vi "Main_FPGA.vi"() -> ()   [LabVIEW 2015]
uses:
  <vilib>/LabVIEW Targets/FPGA/cRIO/shared/nicrio_ModuleControls/nicrio_cRIO-9232_ConfigModeRing.ctl
  <vilib>/rvi/Emulation/niFpgaGetClockAttributes.vi
  <vilib>/rvi/Emulation/niFpgaSctlEmulationGetInTimedLoop.vi
  <vilib>/rvi/Emulation/niFpgaEmulationReportErrorSimple.vi
  <vilib>/rvi/Emulation/niFpgaProcessEmulError.vi
  <vilib>/rvi/eio/common/nirviEmuTemplateMethod_errors.vi
  <vilib>/rvi/interface/RandomDataEmulation/niFpgaRandomDataHandleErrors.vi
  <vilib>/rvi/Emulation/niFpgaCriticalErrorInLSC.vi
  <vilib>/eio/EIONode/EIONode.xnode
  <vilib>/rvi/DataTransferAndStorage/Container/XNode/niFpgaContainer.xnode
  <vilib>/rvi/interface/RandomDataEmulation/nirviRandomDataFpgaReadWriteTemplate.vi
  <vilib>/addons/InsightCM/Devices/Shared/AcquireBOP/FPGA/subVIs/VibAPI/BOP_VibAPI_6.lvlib
panel:
  out "Loop delay (us)":u32
  out "Chassis Temperature":sgl
  in  "Custom Scale Intercept":sgl[](array[numeric])=[0.0, 0.0, 0.0, 0.0, 0.0, 0.0, 0.0, 0.0, 0.0, 0.0, 0.0, 0.0, 0.0, 0.0, 0.0, 0.0, 0.0, 0.0, 0.0, 0.0, 0.0, 0.0, 0.0, 0.0]
  out "FPGA Error":errorcluster
  out "Finished":bool
  in  "Stop":bool
  out "Module Underflow":bool
  out "DMA FIFO Full":bool
  out "Chan Count":bool
  out "Acq Loop Ticks":u32
  out "Short Circuit Chan Array":bool[](array[boolean])
  out "Open Loop Chan Array":bool[](array[boolean])
  out "First Read":bool
  in  "Total Avail Channels":i32=4
  in  "Data Rate [S/s]":u32=1280
  in  "Custom Scale Slope":sgl[](array[numeric])=[0.0, 0.0, 0.0, 0.0, 0.0, 0.0, 0.0, 0.0, 0.0, 0.0, 0.0, 0.0, 0.0, 0.0, 0.0, 0.0, 0.0, 0.0, 0.0, 0.0, 0.0, 0.0, 0.0, 0.0]
  in  "Acquisition Type":enum16{"Finite Samples", "Continuous Samples"}(ring)
  in  "Samps per Chan [Finite]":i32=5120
  in  "Input Config Array":T1[](array[typedef])=[0, 0, 0, 0, 0, 0, 0, 0, 0, 0, 0, 0, 0, 0, 0, 0, 0, 0, 0, 0, 0, 1, 1, 1] items=["AC Coupled", "DC Coupled", "IEPE AC Coupled"]
  in  "Number of Modules":i16=1
  in  "Enable Chan Array":bool[](array[boolean])=[FALSE, FALSE, FALSE, FALSE, FALSE, FALSE, FALSE, FALSE, FALSE, FALSE, FALSE, FALSE, FALSE, FALSE, FALSE, FALSE, FALSE, FALSE, FALSE, FALSE, FALSE, FALSE, FALSE, FALSE]
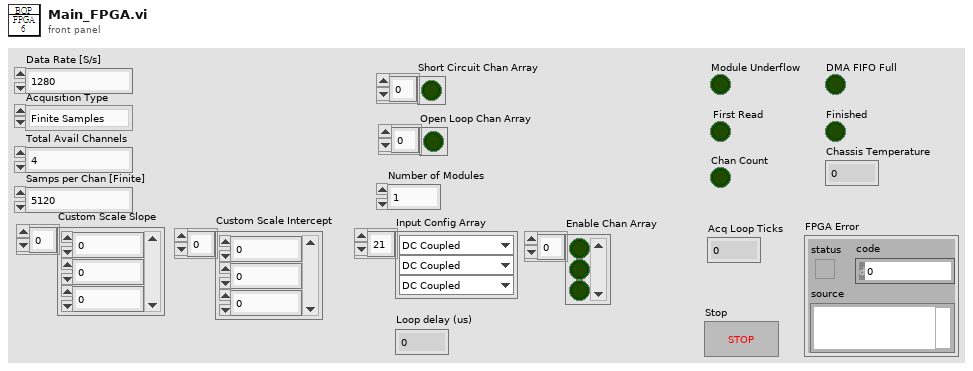
[diagram p1: front panel]
types:
  T1 = typedef "nicrio_cRIO-9232_ConfigModeRing.ctl" = u8
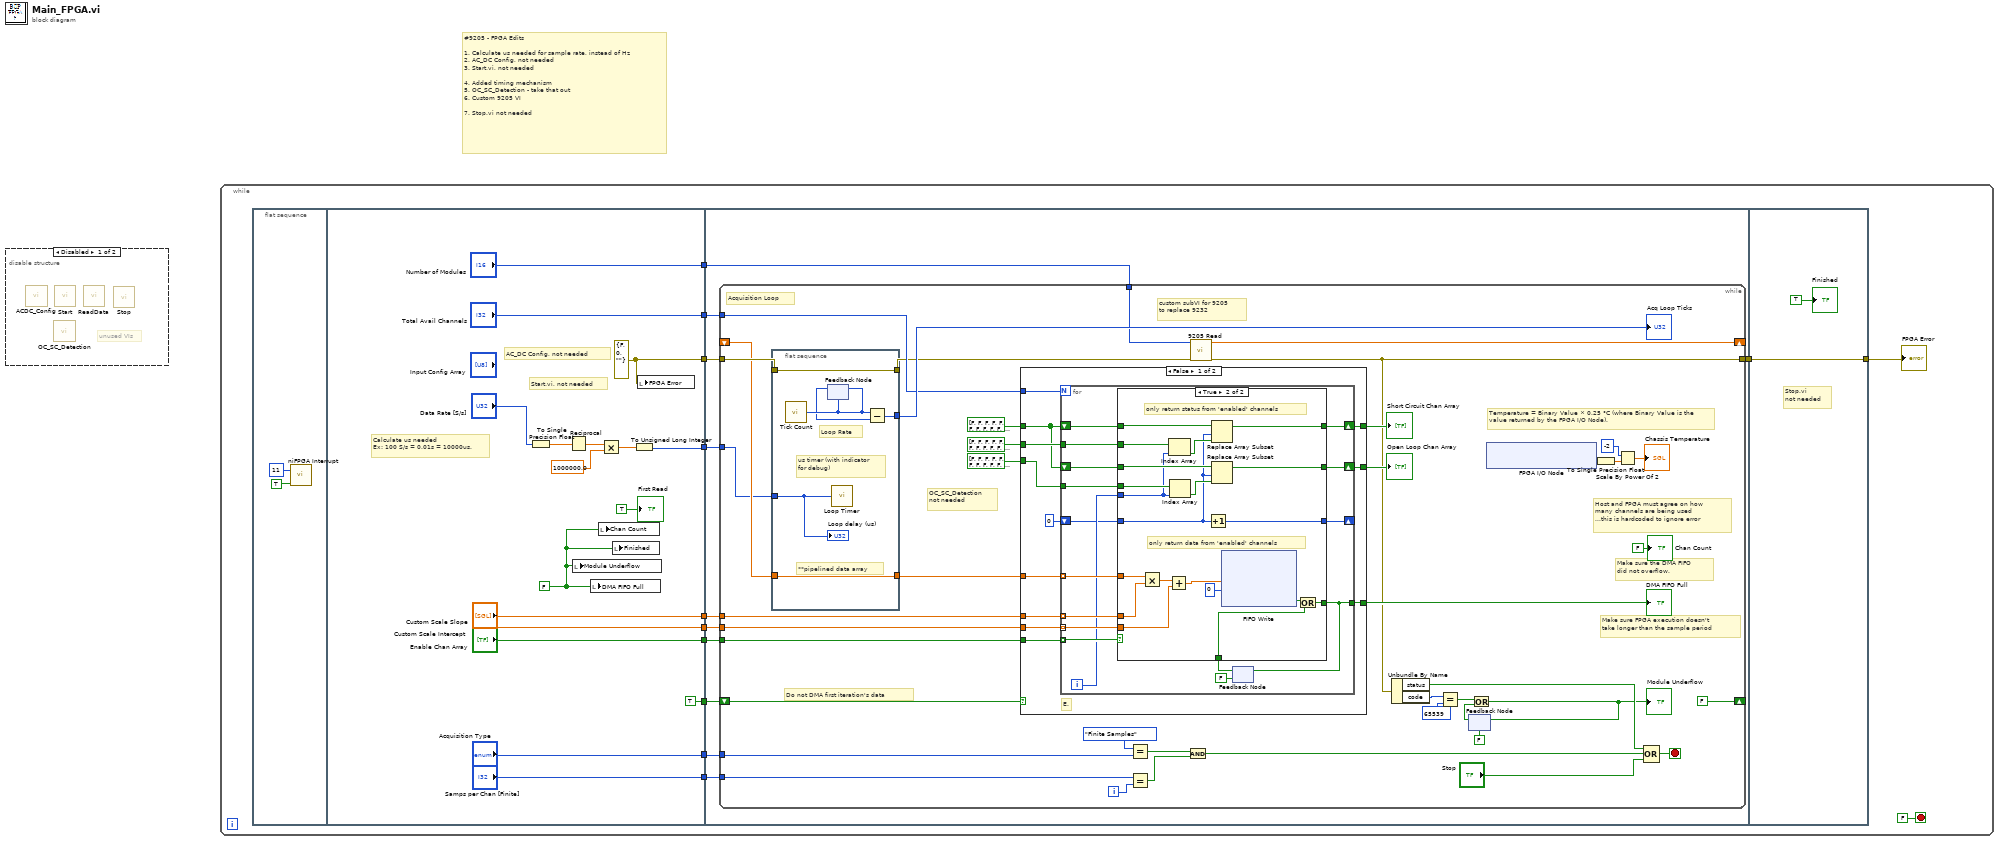
[diagram p0: block diagram]
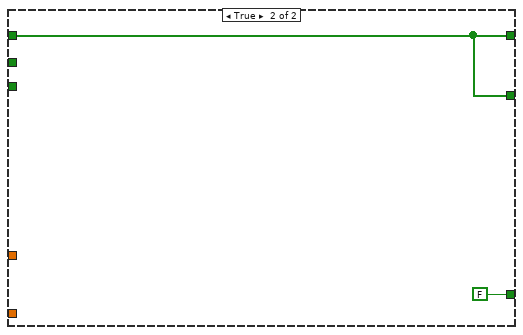
[diagram p4: hidden frame]
diagram:
  # "#9205 - FPGA Edits\n\n1. Calculate us needed for sample rate, instead of Hz\n2. AC_DC Config, not needed\n3. Start.vi, not needed\n\n4. Added timing mechanism\n5. OC_SC_Detection - take that out\n6. Custom 9205 VI\n\n7. Stop.vi not needed"
  n1 = disable-structure shown="Disabled" {
    frame Disabled {
      # "unused VIs"
      n2 = call <vilib>:"ACDC_Config.vi"() -> ()  [unwired: 11 in, 1 out]
      n3 = call <vilib>:"OC_SC_Detection.vi"() -> ()  [unwired: 10 in, 2 out]
      n4 = call <vilib>:"Start.vi"() -> ()  [unwired: 11 in, 1 out]
      n5 = call <vilib>:"ReadData.vi"() -> ()  [unwired: 10 in, 2 out]
      n6 = call <vilib>:"Stop.vi"() -> ()  [unwired: 11 in, 1 out]
    }
    frame Enabled {
    }
  }
  n7 = while {
    stop <- FALSE stop-if-true
    n8 = flat-sequence {
      tunnel: [w22] -> w12
      tunnel: ["Custom Scale Slope"] -> w11
      tunnel: ["Acquisition Type"] -> w10
      tunnel: ["Samps per Chan [Finite]"] -> w9
      tunnel: ["Total Avail Channels"] -> w8
      tunnel: [TRUE ("t")] -> w7
      tunnel: ["Number of Modules"] -> w5
      tunnel: ["Enable Chan Array"] -> w4
      tunnel: ["Custom Scale Intercept"] -> w2
      tunnel: [w16] -> w1
      tunnel: w12 -> [w42]
      tunnel: w11 -> [w41]
      tunnel: w10 -> [w39]
      tunnel: w9 -> [w38]
      tunnel: w8 -> [w43]
      tunnel: w7 -> [w40]
      tunnel: [w37] -> w6
      tunnel: w5 -> [w36]
      tunnel: w4 -> [w35]
      tunnel: w2 -> [w34]
      tunnel: w1 -> [w33]
      tunnel: w6 -> [w146]
      tunnel: [w146] -> w3
      frame #0 {
        n9 = call <vilib>:"niFPGA Interrupt.vi"("Wait Until Cleared (F)"=TRUE ("Wait Until Cleared"), "IRQ Number (0)"=u8 11 ("IRQ Number")) -> ()  [unwired: 1 in]
      }
      frame #1 {
        w22 = errorcluster {"status"=FALSE, "code"=0, "source"=""} ("FPGA Error")
        w27 = FALSE ("Module Underflow")
        # "Start.vi, not needed"
        # "AC_DC Config, not needed"
        # "Calculate us needed\nEx: 100 S/s = 0.01s = 10000us."
        n10 = To Single Precision Float(number="Data Rate [S/s]") -> (single precision float=w19:sgl)
        n11 = Reciprocal(x=w19) -> (1/x=w21:sgl)
        n12 = local write "Module Underflow"(w27) -> ()
        n13 = local write "DMA FIFO Full"(w27) -> ()
        n14 = local write "Chan Count"(w27) -> ()
        n15 = Multiply(x=w21, y=sgl 1000000.0) -> (x*y=w17:sgl)
        n16 = local write "Finished"(w27) -> ()
        n17 = To Unsigned Long Integer(number=w17) -> (unsigned 32bit integer=w16:u32)
        n18 = local write "FPGA Error"(w22) -> ()
        "First Read" <- TRUE ("First Read")
      }
      frame #2 {
        n19 = while {
          tunnel: w42 -> [w79]
          tunnel: [w46] -> w37
          tunnel: w39 -> [w81]
          tunnel: w38 -> [w80]
          shift-right: [w44] -> _
          shift-left: _ -> [w77]
          tunnel: w43 -> [w61]
          tunnel: w41 -> [w60]
          shift-right: [FALSE ("t")] -> _
          shift-left: w40 -> [w64]
          tunnel: w36 -> [w45]
          tunnel: w35 -> [w59]
          tunnel: w34 -> [w58]
          tunnel: w33 -> [w50]
          i -> [w75]
          stop <- w84 stop-if-true
          # "custom subVI for 9205\nto replace 9232"
          # "OC_SC_Detection\nnot needed"
          # "Temperature = Binary Value × 0.25 °C (where Binary Value is the value returned by the FPGA I/O Node)."
          # "Do not DMA first iteration's data"
          # "Acquisition Loop"
          # "Host and FPGA must agree on how \nmany channels are being used\n...this is hardcoded to ignore error"
          # "Make sure the DMA FIFO\ndid not overflow."
          # "Make sure FPGA execution doesn't\ntake longer than the sample period"
          n20 = flat-sequence {
            tunnel: [w145] -> w47
            tunnel: w79 -> [w145]
            tunnel: [w142] -> w78
            tunnel: w77 -> [w141]
            tunnel: [w141] -> w62
            tunnel: w50 -> [w140]
            frame #0 {
              # "us timer (with indicator\nfor debug)"
              # "**pipelined data array"
              # "Loop Rate"
              n21 = call "Tick Count"() -> ("Tick Count(Ticks)"=w144:u32)
              n22 = feedback-in #1(w144) -> ()
              n23 = feedback #1(w144) -> (w143:u32)
              n24 = call "Loop Timer"("Count(uSec)"=w140) -> ()  [unwired: 1 out]
              n25 = Subtract(x=w144, y=w143) -> (x-y=w142:u32)
              "Loop delay (us)" <- w140
            }
          }
          n26 = case shown="False" w64 {
            tunnel: [w97 FALSE] -> w63
            tunnel: w60 -> [w96 _]
            tunnel: w62 -> [w95 _]
            tunnel: w61 -> [w94 _]
            tunnel: w59 -> [w93 _]
            tunnel: w58 -> [w92 _]
            tunnel: bool[] [FALSE, FALSE, FALSE, FALSE, FALSE, FALSE, FALSE, FALSE, FALSE, FALSE, FALSE, FALSE, FALSE, FALSE, FALSE, FALSE, FALSE, FALSE, FALSE, FALSE, FALSE, FALSE, FALSE, FALSE] ("Short Circuit Channels Array") -> [w91 _]
            tunnel: bool[] [FALSE, FALSE, FALSE, FALSE, FALSE, FALSE, FALSE, FALSE, FALSE, FALSE, FALSE, FALSE, FALSE, FALSE, FALSE, FALSE, FALSE, FALSE, FALSE, FALSE, FALSE, FALSE, FALSE, FALSE] ("Open Loop Channels Array") -> [w90 _]
            tunnel: bool[] [FALSE, FALSE, FALSE, FALSE, FALSE, FALSE, FALSE, FALSE, FALSE, FALSE, FALSE, FALSE, FALSE, FALSE, FALSE, FALSE, FALSE, FALSE, FALSE, FALSE, FALSE, FALSE, FALSE, FALSE] ("Open Loop Chan Array") -> [w89 w138]
            tunnel: [w88 w138] -> w56
            tunnel: [w87 w138] -> w55
            frame False {
              # "E."
              n27 = for {
                N: w94 -> [_]
                tunnel: [w112] -> w97
                tunnel: w95 -> [w111] mode=indexing
                tunnel: w96 -> [w110] mode=indexing
                tunnel: w93 -> [w108] mode=indexing
                tunnel: w92 -> [w107] mode=indexing
                tunnel: w91 -> [w101]
                tunnel: w90 -> [w102]
                shift-right: [w104] -> w88
                shift-left: w89 -> [w105]
                shift-right: [w103] -> w87
                shift-left: w89 -> [w106]
                shift-right: [w98] -> _
                shift-left: 0 -> [w99]
                i -> [w100]
                n28 = feedback #2(FALSE) -> (w113:bool)
                n29 = case shown="True" w108 {
                  tunnel: w113 -> [w117 w137]
                  tunnel: [w117 w136] -> w112
                  tunnel: w111 -> [_ w135]
                  tunnel: w110 -> [_ w134]
                  tunnel: w107 -> [_ w129]
                  tunnel: w106 -> [w115 w126]
                  tunnel: w105 -> [w116 w125]
                  tunnel: [w116 w124] -> w104
                  tunnel: [w115 w123] -> w103
                  tunnel: w102 -> [_ w122]
                  tunnel: w101 -> [_ w121]
                  tunnel: w100 -> [_ w120]
                  tunnel: w99 -> [w114 w119]
                  tunnel: [w114 w118] -> w98
                  frame False {
                  }
                  frame True {
                    # "only return status from 'enabled' channels"
                    # "only return data from 'enabled' channels"
                    n30 = Multiply(x=w135, y=w134) -> (x*y=w131:sgl)
                    n31 = Add(x=w131, y=w129) -> (x+y=w130:sgl)
                    n32 = Index Array(array=w121, index=w120) -> (element=w128:bool)
                    n33 = Index Array(array=w122, index=w120) -> (element=w127:bool)
                    n34 = Increment(x=w119) -> (x+1=w118:i32)
                    n35 = Replace Array Subset(array=w125, new element=w128, index=w119) -> (w124:bool[])
                    n36 = Replace Array Subset(array=w126, new element=w127, index=w119) -> (w123:bool[])
                    n37 = xnode ("FIFO Write")("Element"=w130, "Timeout"=0) -> ("Timed Out?"=w132:bool)  [unwired: 1 in, 1 out]
                    n38 = Or(x=w132, y=w137) -> (x .or. y?=w136:bool)
                  }
                }
                n39 = feedback-in #2(w112) -> ()
              }
            }
            frame True {
            }
          }
          "DMA FIFO Full" <- w63
          "Short Circuit Chan Array" <- w56
          "Open Loop Chan Array" <- w55
          n40 = Equal?(x=enum16{"Finite Samples", "Continuous Samples"}."Finite Samples" ("y"), y=w81) -> (x = y?=w69:bool)
          n41 = Equal?(x=w80, y=w75) -> (x = y?=w68:bool)
          n42 = And(x=w69, y=w68) -> (x .and. y?=w67:bool)
          n43 = call "9205 Read.vi"("error in"=w47, "Module Config Selector"=w45) -> ("error out"=w46:errorcluster, "Data Array"=w44:sgl[])  [unwired: 8 in]
          n44 = Unbundle By Name(w46) -> ("status"=w74:bool, "code"=w82:i32)
          n45 = Equal?(x=w82, y=65539) -> (x = y?=w71:bool)
          n46 = feedback #3(FALSE) -> (w73:bool)
          n47 = Or(x=w71, y=w73) -> (x .or. y?=w70:bool)
          "Module Underflow" <- w70
          n48 = feedback-in #3(w70) -> ()
          n49 = xnode "FPGA I/O Node"() -> ("Chassis Temperature"=w52:i16)  [unwired: 1 in, 1 out]
          n50 = To Single Precision Float(number=w52) -> (single precision float=w54:sgl)
          n51 = Scale By Power Of 2(n=i16 -2, x=w54) -> (x*2^n=→"Chassis Temperature":sgl)
          n52 = Compound Arithmetic op=OR(w74, w67, "Stop") -> (w84:bool)
          "Chan Count" <- FALSE ("Chan Count")
          "Acq Loop Ticks" <- w78
        }
      }
      frame #3 {
        # "Stop.vi\nnot needed"
        "Finished" <- TRUE ("Finished")
      }
    }
    "FPGA Error" <- w3
  }
